vi "ALTS-2015 Clear OPC Write Data.vi"(8 "error in (no error)":errorcluster) -> (0 "error out":errorcluster)   [LabVIEW 2013]
uses:
  OPC Engine/Controls/ALTS-2015 OPC Write Global Options.ctl
  OPC Engine/Controls/ALTS-2015 OPC Write Registers.ctl
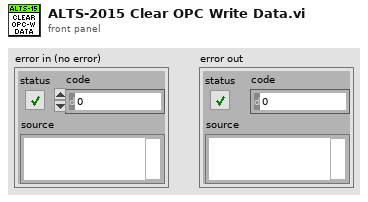
[diagram p1: front panel]
types:
  T1 = typedef "ALTS-2015 OPC Write Registers.ctl" = enum16{"Task_Available_for_Robot", "New_Serial", "Serial_Adapter_Size", "Serial_Displacement_Size", "Serial_Flange_Size", "Serial_Height", "Serial_LoadDecision", "Serial_CartInsert", "Test_Result", "Station_Number", "Rerun", "Invalid_SNo", "PC_ACK_Read_Tags", "No_Test"}
  T2 = typedef "ALTS-2015 OPC Write Global Options.ctl" = enum16{"Init", "Write Value", "Write Array", "Read Value", "Read Array", "Read All"}
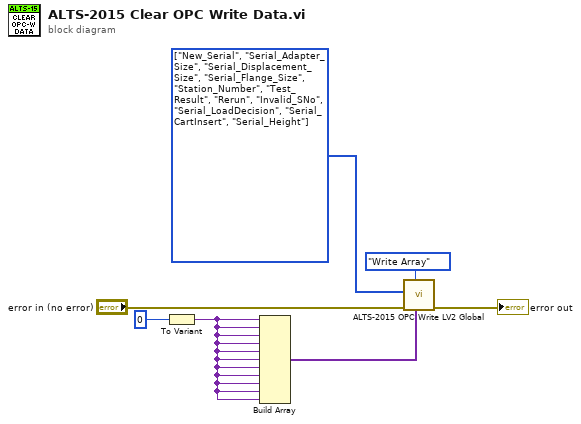
[diagram p0: block diagram]
diagram:
  w7 = T1[] [enum."New_Serial", enum."Serial_Adapter_Size", enum."Serial_Displacement_Size", enum."Serial_Flange_Size", enum."Station_Number", enum."Test_Result", enum."Rerun", enum."Invalid_SNo", enum."Serial_LoadDecision", enum."Serial_CartInsert", enum."Serial_Height"] items=["Task_Available_for_Robot", "New_Serial", "Serial_Adapter_Size", "Serial_Displacement_Size", "Serial_Flange_Size", "Serial_Height", "Serial_LoadDecision", "Serial_CartInsert", "Test_Result", "Station_Number", "Rerun", "Invalid_SNo", "PC_ACK_Read_Tags", "No_Test"] ("OPC Write Register Array")
  n1 = To Variant(anything=i16 0) -> (Variant=w1:variant)
  n2 = Build Array(w1, w1, w1, w1, w1, w1, w1, w1, w1, w1, w1) -> (w6:variant[])
  n3 = call "ALTS-2015 OPC Write LV2 Global.vi"("OPC value Array"=w6, "Options"=ALTS-2015_OPC_Write_Global_Options."Write Array", "error in (no error)"="error in (no error)", "OPC Write Register Array"=w7) -> ("error out"=→"error out":errorcluster)  [unwired: 5 in, 2 out]
